vi "X10control.vi"(0 "Port Name":string, 2 "Power Request (ON)":bool, 3 "House Code":i32(ring)=1 items=["-----", "A", "B", "C", "D", "E", "F", "G", "H", "I", "J", "K", "L", "M", "N", "O", "P"], 4 "Unit No.":i32=1 min=1 max=16) -> ()   [LabVIEW 2010]
panel:
  out "Read String":string
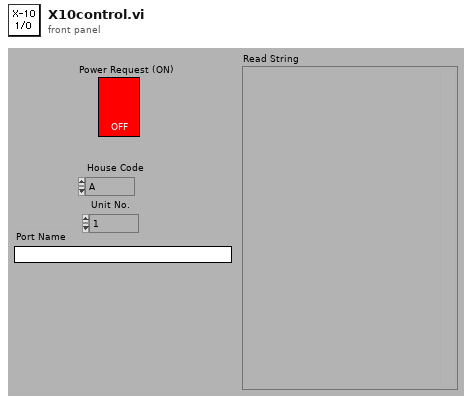
[diagram p1: front panel]
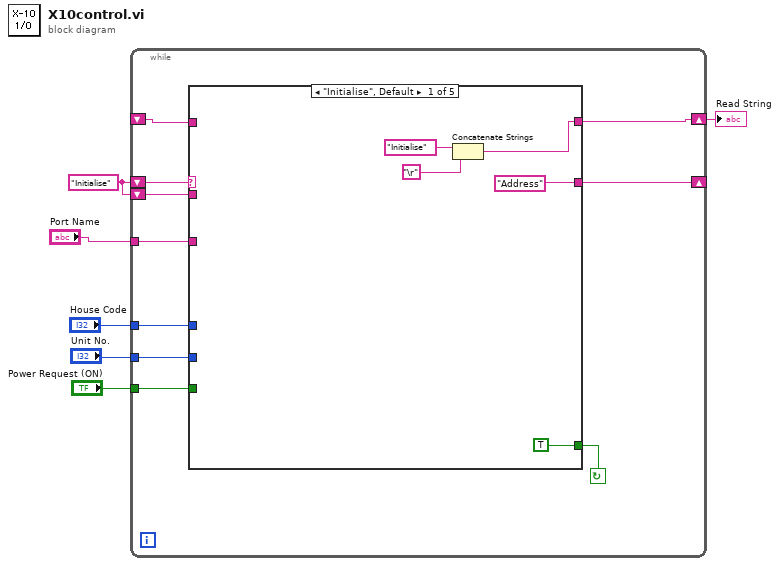
[diagram p0: block diagram]
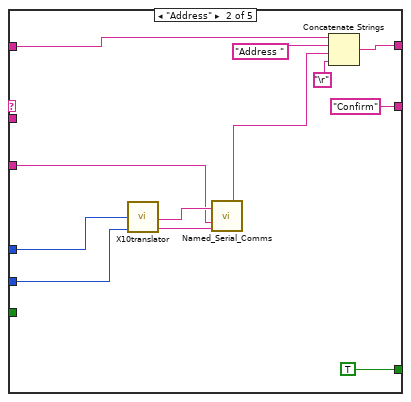
[diagram p2: hidden frame]
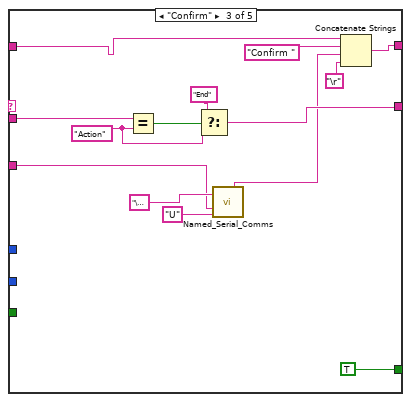
[diagram p3: hidden frame]
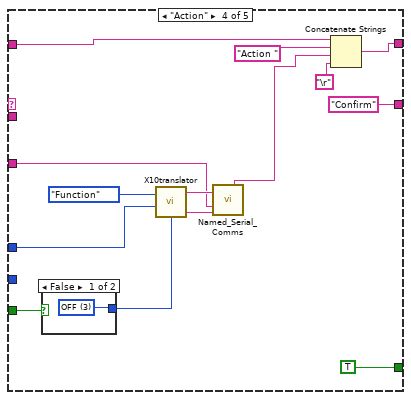
[diagram p4: hidden frame]
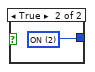
[diagram p5: hidden frame]
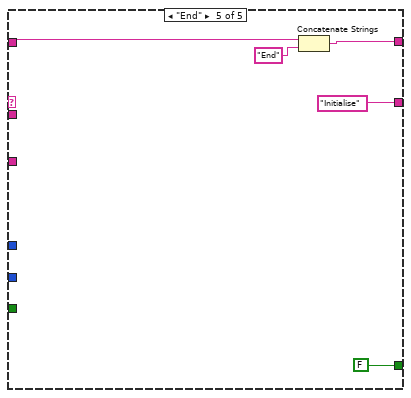
[diagram p6: hidden frame]
diagram:
  w3 = "Initialise"
  n1 = while {
    shift-left: w3 -> [w9]
    tunnel: "House Code" -> [w12]
    tunnel: "Unit No." -> [w13]
    tunnel: "Power Request (ON)" -> [w14]
    shift-left: w3 -> [w11]
    shift-right: [w10] -> _
    tunnel: "Port Name" -> [w16]
    shift-right: [w7] -> w1
    shift-left: _ -> [w8]
    stop <- w15 continue-if-true
    n2 = case shown="\"Initialise\", Default" w11 {
      tunnel: w16 -> [_ w27 w39 w53 _]
      tunnel: [TRUE TRUE TRUE TRUE FALSE] -> w15
      tunnel: w14 -> [_ _ _ w60 _]
      tunnel: w13 -> [_ w30 _ _ _]
      tunnel: w12 -> [_ w29 _ w55 _]
      tunnel: ["Address" "Confirm" w42 "Confirm" "Initialise"] -> w10
      tunnel: w9 -> [_ _ w44 _ _]
      tunnel: w8 -> [_ w24 w36 w49 w66]
      tunnel: [w17 w23 w35 w50 w65] -> w7
      frame "Initialise", Default {
        n3 = Concatenate Strings("Initialise" ("string"), "\r") -> (w17:string)
      }
      frame "Address" {
        n4 = call "X10translator.vi"("Unit No."=w30, "House Code"=w29) -> ("checksum"=w32:string, "Send string"=w31:string)  [unwired: 4 in]
        n5 = call "Named_Serial_Comms.vi"("Write String"=w31, "Port Name"=w27, "Term Grep"=w32) -> ("Read"=w25:string)  [unwired: 6 in, 6 out]
        n6 = Concatenate Strings(w24, "Address ", w25, "\r") -> (w23:string)
      }
      frame "Confirm" {
        w40 = "Action"
        n7 = Equal?(x=w44, y=w40) -> (x = y?=w43:bool)
        n8 = Select(t="End" ("f"), s=w43, f=w40) -> (s? t:f=w42:string)
        n9 = call "Named_Serial_Comms.vi"("Write String"="\u0000" ("string to write"), "Port Name"=w39, "Term Grep"="U" ("string to write")) -> ("Read"=w34:string)  [unwired: 6 in, 6 out]
        n10 = Concatenate Strings(w36, "Confirm ", w34, "\r") -> (w35:string)
      }
      frame "Action" {
        n11 = case shown="False" w60 {
          tunnel: [w62 w63] -> w56
          frame False {
            w62 = u8 3 items=["All lights OFF", "All lights ON", "ON", "OFF", "Dim", "Bright", "All lights OFF", "Extended Code", "Hail Request", "Hail Acknowledge", "Pre-set Dim (1)", "Pre-set Dim (2)", "Extended data transfer", "Status ON", "Status OFF", "Status Request"] ("Function Codes (ON)")
          }
          frame True {
            w63 = u8 2 items=["All lights OFF", "All lights ON", "ON", "OFF", "Dim", "Bright", "All lights OFF", "Extended Code", "Hail Request", "Hail Acknowledge", "Pre-set Dim (1)", "Pre-set Dim (2)", "Extended data transfer", "Status ON", "Status OFF", "Status Request"] ("Function Codes (ON)")
          }
        }
        n12 = call "X10translator.vi"("House Code"=w55, "Function Codes (ON)"=w56, "Transmission type (address)"=enum8{"Address", "Function"}."Function") -> ("checksum"=w58:string, "Send string"=w59:string)  [unwired: 3 in]
        n13 = call "Named_Serial_Comms.vi"("Write String"=w59, "Port Name"=w53, "Term Grep"=w58) -> ("Read"=w48:string)  [unwired: 6 in, 6 out]
        n14 = Concatenate Strings(w49, "Action ", w48, "\r") -> (w50:string)
      }
      frame "End" {
        n15 = Concatenate Strings(w66, "End" ("string")) -> (w65:string)
      }
    }
  }
  "Read String" <- w1
